vi "Configure Histogram.vi"(4 "Lower Range (0)":dbl, 5 "Upper Range (0)":dbl, 6 "Auto Selection Number (100)":i32=100, 7 "Point Number (100)":i32=100, 8 "error in (no error)":errorcluster, 9 "Enable Automatic Selection (T: Enable)":bool=TRUE, 10 "Enable Histogram Computation (T: Enable)":bool=TRUE, 11 "VISA resource name":refnum<visa-resource-name>) -> (0 "error out":errorcluster, 3 "VISA resource name out":refnum<visa-resource-name>)   [LabVIEW 2021, in "Agilent 532XX Series.lvlib"]
doc: "Configures the parameters required for histogram computation"
uses:
  <instrlib>/Agilent 532XX Series/Agilent 532XX Series.lvlib
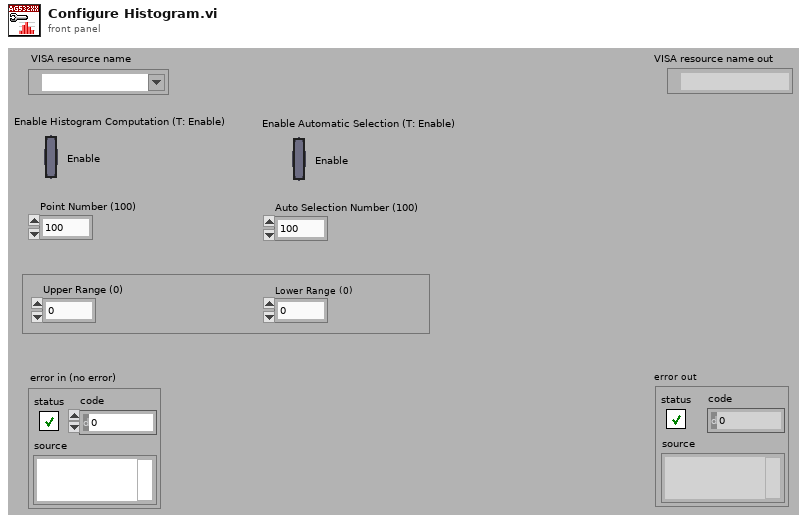
[diagram p1: front panel]
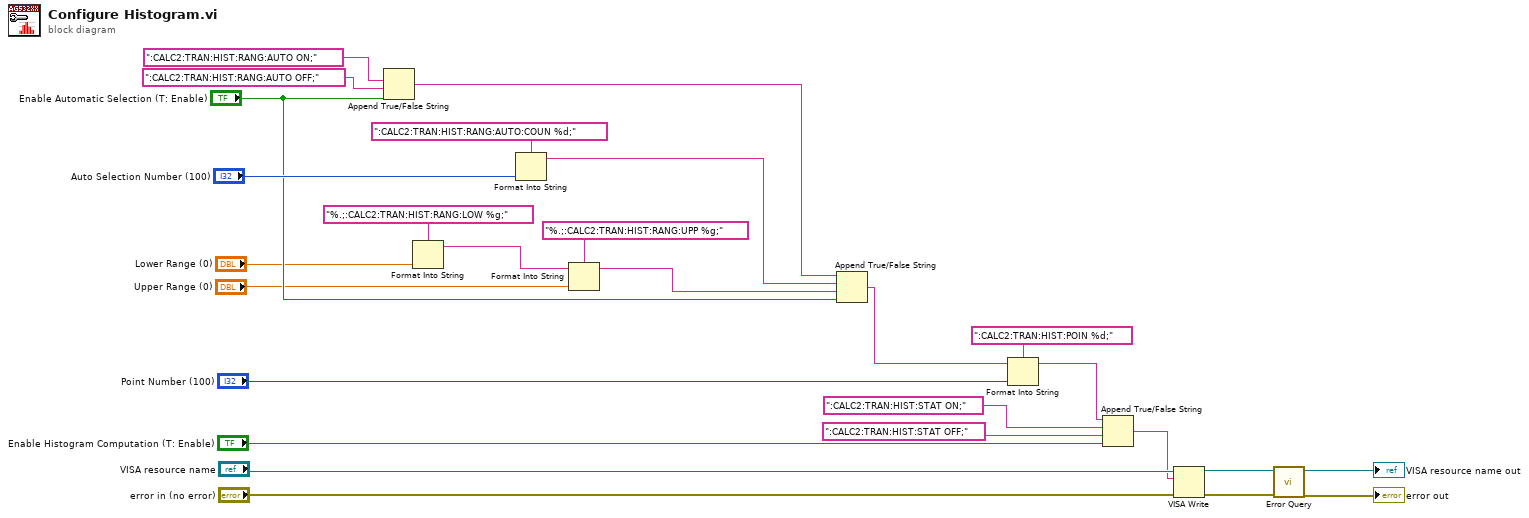
[diagram p0: block diagram]
diagram:
  n1 = Append True/False String(1:"Enable Automatic Selection (T: Enable)", 2:":CALC2:TRAN:HIST:RANG:AUTO OFF;", 3:":CALC2:TRAN:HIST:RANG:AUTO ON;") -> (0:w4:string)  [unwired: 1 out]
  n2 = Format Into String(format string="%.;:CALC2:TRAN:HIST:RANG:LOW %g;", "Lower Range (0)") -> (resulting string=w6:string)  [unwired: 2 in, 1 out]
  n3 = Format Into String(format string=":CALC2:TRAN:HIST:RANG:AUTO:COUN %d;", "Auto Selection Number (100)") -> (resulting string=w5:string)  [unwired: 2 in, 1 out]
  n4 = Format Into String(format string="%.;:CALC2:TRAN:HIST:RANG:UPP %g;", initial string=w6, "Upper Range (0)") -> (resulting string=w7:string)  [unwired: 1 in, 1 out]
  n5 = Append True/False String(1:"Enable Automatic Selection (T: Enable)", 2:w7, 3:w5, 4:w4) -> (0:w3:string)
  n6 = Format Into String(format string=":CALC2:TRAN:HIST:POIN %d;", initial string=w3, "Point Number (100)") -> (resulting string=w23:string)  [unwired: 1 in, 1 out]
  n7 = Append True/False String(1:"Enable Histogram Computation (T: Enable)", 2:":CALC2:TRAN:HIST:STAT OFF;", 3:":CALC2:TRAN:HIST:STAT ON;", 4:w23) -> (0:w13:string)
  n8 = VISA Write(VISA resource name="VISA resource name", write buffer=w13, error in (no error)="error in (no error)") -> (VISA resource name out=w19:refnum<visa-resource-name>, error out=w18:errorcluster)  [unwired: 1 out]
  n9 = call <instrlib>:"Error Query.vi"("error in (no error)"=w18, "VISA resource name"=w19) -> ("error out"=→"error out":errorcluster, "VISA resource name out"=→"VISA resource name out":refnum<visa-resource-name>)  [unwired: 8 out]
